vi "test_auto.vi"   [LabVIEW 2012, in "Test.lvrbt"]
uses:
  Test.lvrbt
  <vilib>/NXT/LegoClasses/BrickReference/BrickReference.lvclass
  <vilib>/NXT/Subs/LVHSConnector.ctl
  <vilib>/NXT/NXTIO Xnodes/NXTIOXNode/NXTIO.xnode
  <vilib>/NXT/Hardware/Plugins/Tetrix DC Motor/TetrixDCMotorAddress.ctl
  <vilib>/NXT/NXTIO Xnodes/AddressXNode/NXTIOAddress.xnode
  <vilib>/NXT/NXTIO Xnodes/NXTIONodeSubVIs/TETRIX IO Move DC Motors.vi
  <vilib>/NXT/Dual Mode Library/Waits/Wait_Num.vi
  <vilib>/NXT/NXTIO Xnodes/NXTIONodeSubVIs/TETRIX IO Stop DC Motors.vi
types:
  T1 = typedef "LVHSConnector.ctl" = refnum<class "BrickReference.lvclass">
  T2 = typedef "TetrixDCMotorAddress.ctl" = i32
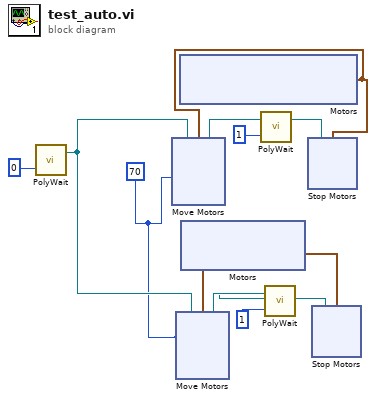
[diagram p0: block diagram]
diagram:
  w1 = 70
  n1 = call-poly <vilib>:"PolyWait.vi"("Time (1 sec)"=0) -> ("NXT/EV3"=w7:T1)  [unwired: 3 in]
  n2 = xnode ("Motors")() -> ("Motor"=w2:cluster{"TetrixDCMotor":T2, "TetrixDCMotor":T2})
  n3 = xnode ("Move Motors")("Power/Speed 2"=w1, "Power/Speed 1"=w1, "Motors"=w2, "NXT/EV3"=w7) -> ("NXT/EV3"=w9:T1)
  n4 = xnode ("Motors")() -> ("Motor"=w3:cluster{"TetrixDCMotor":T2, "TetrixDCMotor":T2})
  n5 = xnode ("Move Motors")("Power/Speed 2"=w1, "Power/Speed 1"=w1, "Motors"=w3, "NXT/EV3"=w7) -> ("NXT/EV3"=w5:T1)
  n6 = call-poly <vilib>:"PolyWait.vi"("Time (1 sec)"=1, "NXT/EV3"=w9) -> ("NXT/EV3"=w10:T1)  [unwired: 2 in]
  n7 = call-poly <vilib>:"PolyWait.vi"("Time (1 sec)"=1, "NXT/EV3"=w5) -> ("NXT/EV3"=w4:T1)  [unwired: 2 in]
  n8 = xnode "Stop Motors"("Motors"=w2, "NXT/EV3"=w10) -> ()  [unwired: 1 out]
  n9 = xnode "Stop Motors"("Motors"=w3, "NXT/EV3"=w4) -> ()  [unwired: 1 out]
